vi "DC Supply Configure.vi"(0 "VISA resource name":refnum<visa-resource-name>, 5 "Voltage(0 Volts)":dbl format="%.3f", 7 "Current(0 Amps)":dbl format="%.3f", 11 "error in":errorcluster, 12 "Protection(None:0)":u16(ring) items=["None", "Overcurrent protection", "Overvoltage protection", "Overcurrent and overvoltage protection", "Clear overvoltage condition", "Clear overcurrent protection", "Set time delay"], 13 "Overvoltage prot value":dbl=9.0 caption="Overvoltage prot value (9 Volts)" format="%.3f", 14 "Time Delay(0 seconds)":dbl format="%.4f") -> (4 "VISA resource name out":refnum<visa-resource-name>, 15 "error out":errorcluster)   [LabVIEW 2019, in "DAC.lvlib" / "DAC DC Supply.lvclass"]
uses:
  DAC DC Supply.lvclass
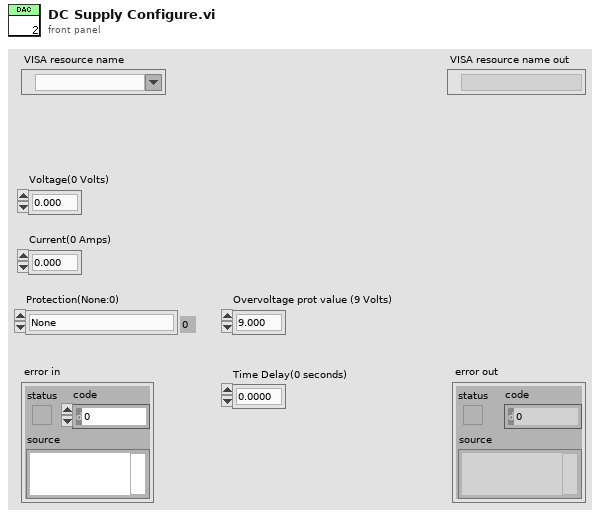
[diagram p1: front panel]
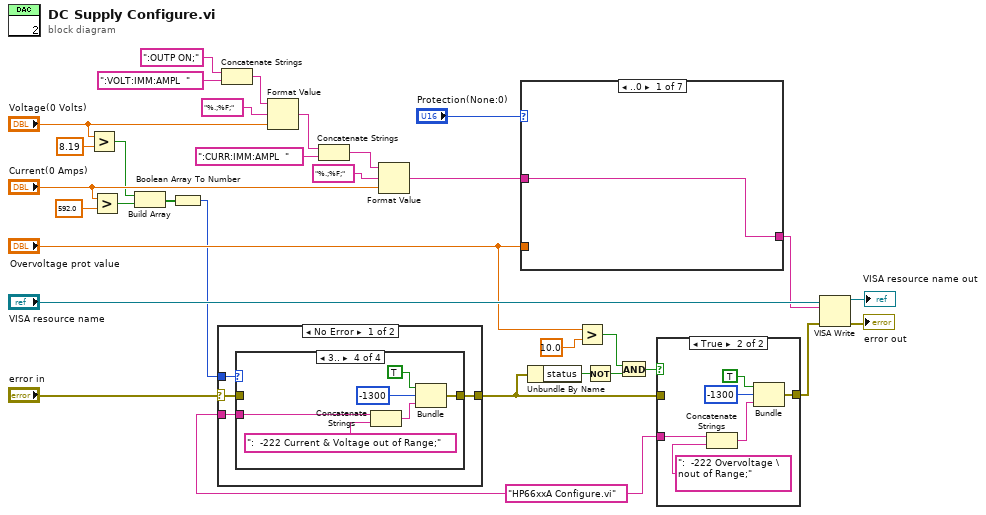
[diagram p0: block diagram]
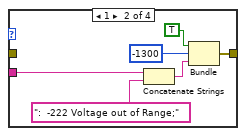
[diagram p4: hidden frame]
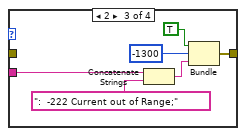
[diagram p5: hidden frame]
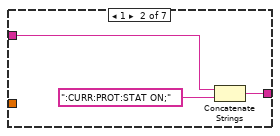
[diagram p7: hidden frame]
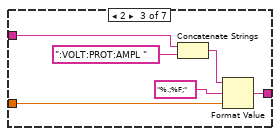
[diagram p8: hidden frame]
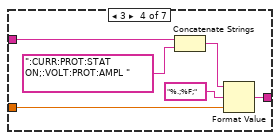
[diagram p9: hidden frame]
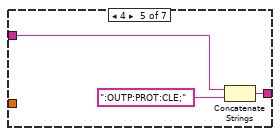
[diagram p10: hidden frame]
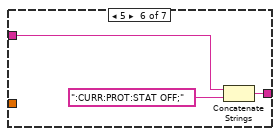
[diagram p11: hidden frame]
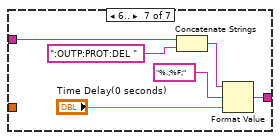
[diagram p12: hidden frame]
diagram:
  w13 = "HP66xxA Configure.vi"
  n1 = Greater?(x="Voltage(0 Volts)", y=8.19) -> (0:w21:bool)
  n2 = Greater?(x="Current(0 Amps)", y=592.0) -> (0:w20:bool)
  n3 = Build Array(w21, w20) -> (w19:bool[])
  n4 = Boolean Array To Number(Boolean array=w19) -> (number=w18:u32)
  n5 = case shown="No Error" "error in" {
    selector: "error in" -> [w33 w56]
    tunnel: [w36 w56] -> w16
    tunnel: w13 -> [w35 _]
    tunnel: w18 -> [w34 _]
    frame No Error {
      n6 = case shown="3.." w34 {
        tunnel: [w37 w38 w44 w50] -> w36
        tunnel: w35 -> [_ w39 w45 w51]
        tunnel: w33 -> [w37 _ _ _]
        frame ..0 {
        }
        frame 1 {
          n7 = Concatenate Strings(w39, ":  -222 Voltage out of Range;") -> (w40:string)
          n8 = Bundle(TRUE, -1300, w40) -> (w38:errorcluster)  [unwired: 1 in]
        }
        frame 2 {
          n9 = Concatenate Strings(w45, ":  -222 Current out of Range;") -> (w46:string)
          n10 = Bundle(TRUE, -1300, w46) -> (w44:errorcluster)  [unwired: 1 in]
        }
        frame 3.. {
          n11 = Concatenate Strings(w51, ":  -222 Current & Voltage out of Range;") -> (w52:string)
          n12 = Bundle(TRUE, -1300, w52) -> (w50:errorcluster)  [unwired: 1 in]
        }
      }
    }
    frame Error {
    }
  }
  n13 = Concatenate Strings(":OUTP ON;", ":VOLT:IMM:AMPL  ") -> (w10:string)
  n14 = Format Value(string ("")=w10, format string="%.;%F;", value (0)="Voltage(0 Volts)") -> (output string=w9:string)
  n15 = Concatenate Strings(w9, ":CURR:IMM:AMPL  ") -> (w7:string)
  n16 = Format Value(string ("")=w7, format string="%.;%F;", value (0)="Current(0 Amps)") -> (output string=w29:string)
  n17 = case shown="..0" "Protection(None:0)" {
    tunnel: w29 -> [w57 w60 w66 w69 w75 w77 w84]
    tunnel: [w57 w58 w62 w70 w73 w76 w79] -> w24
    tunnel: "Overvoltage prot value" -> [_ _ w61 w67 _ _ _]
    frame ..0 {
    }
    frame 1 {
      n18 = Concatenate Strings(w60, ":CURR:PROT:STAT ON;") -> (w58:string)
    }
    frame 2 {
      n19 = Concatenate Strings(w66, ":VOLT:PROT:AMPL ") -> (w64:string)
      n20 = Format Value(string ("")=w64, format string="%.;%F;", value (0)=w61) -> (output string=w62:string)
    }
    frame 3 {
      n21 = Concatenate Strings(w69, ":CURR:PROT:STAT ON;:VOLT:PROT:AMPL ") -> (w72:string)
      n22 = Format Value(string ("")=w72, format string="%.;%F;", value (0)=w67) -> (output string=w70:string)
    }
    frame 4 {
      n23 = Concatenate Strings(w75, ":OUTP:PROT:CLE;") -> (w73:string)
    }
    frame 5 {
      n24 = Concatenate Strings(w77, ":CURR:PROT:STAT OFF;") -> (w76:string)
    }
    frame 6.. {
      n25 = Concatenate Strings(w84, ":OUTP:PROT:DEL ") -> (w81:string)
      n26 = Format Value(string ("")=w81, format string="%.;%F;", value (0)="Time Delay(0 seconds)") -> (output string=w79:string)
    }
  }
  n27 = Unbundle By Name(w16) -> ("status"=w15:bool)
  n28 = Greater?(x="Overvoltage prot value", y=10.0) -> (0:w1:bool)
  n29 = Not(x=w15) -> (.not. x?=w2:bool)
  n30 = And(x=w1, y=w2) -> (x .and. y?=w14:bool)
  n31 = case shown="True" w14 {
    tunnel: w13 -> [_ w87]
    tunnel: w16 -> [w85 _]
    tunnel: [w85 w86] -> w17
    frame False {
    }
    frame True {
      n32 = Concatenate Strings(w87, ":  -222 Overvoltage \nout of Range;") -> (w88:string)
      n33 = Bundle(TRUE, -1300, w88) -> (w86:errorcluster)  [unwired: 1 in]
    }
  }
  n34 = VISA Write(VISA resource name="VISA resource name", write buffer=w24, error in (no error)=w17) -> (VISA resource name out=→"VISA resource name out":refnum<visa-resource-name>, error out=→"error out":errorcluster)  [unwired: 1 out]
